vi "Retrieve Number Of Processors From Registry.vi"(8 "error in":errorcluster) -> (0 "error out":errorcluster, 3 "Number Of Cores":i32)   [LabVIEW 2013, in "Win32 Util.lvlib"]
doc: "Query the Windows registry for the number of processors present in the system.\n\nNote: this VI has not been thoroughly tested. It works fine on the developers Quad core."
uses:
  Win32 Util.lvlib
  <vilib>/registry/registry.llb/Registry SAM.ctl
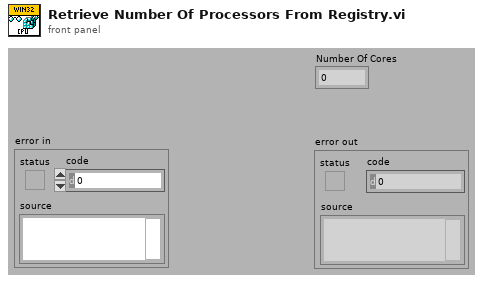
[diagram p1: front panel]
types:
  T1 = typedef "Registry SAM.ctl" = enum32{"KEY_QUERY_VALUE", "KEY_SET_VALUE", "KEY_CREATE_SUB_KEY", "KEY_ENUMERATE_SUB_KEYS", "KEY_NOTIFY", "KEY_CREATE_LINK", "KEY_READ", "KEY_WRITE", "KEY_ALL_ACCESS", "KEY_READ | KEY_WRITE"}
  T2 = typedef "Registry refnum.ctl" = refnum<k1>
  T3 = cluster{"numSubKeys":i32, "maxSubKeyLen":i32, "maxSubKeyClassLen":i32}
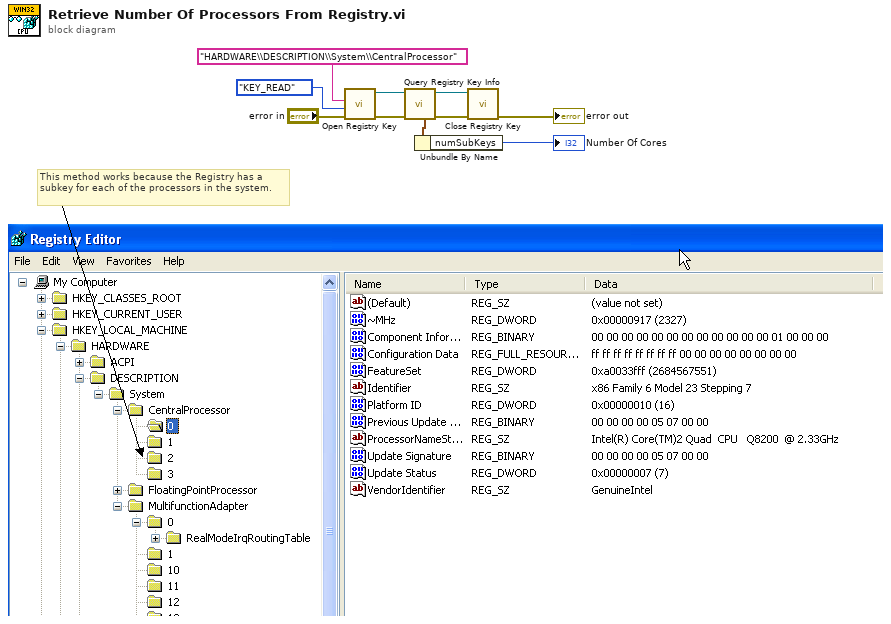
[diagram p0: block diagram]
diagram:
  # "This method works because the Registry has a subkey for each of the processors in the system."
  n1 = call <vilib>:"Open Registry Key.vi"("error in (no error)"="error in", "security access mask (KEY_READ | KEY_WRITE)"=Registry_SAM."KEY_READ", "subkey"="HARDWARE\\DESCRIPTION\\System\\CentralProcessor") -> ("error out"=w6:errorcluster, "refnum out"=w9:T2)  [unwired: 1 in, 6 out]
  n2 = call <vilib>:"Query Registry Key Info.vi"("error in (no error)"=w6, "refnum"=w9) -> ("error out"=w5:errorcluster, "refnum out"=w8:T2, "subkey info"=w7:T3)  [unwired: 7 out]
  n3 = Unbundle By Name(w7) -> ("numSubKeys"=→"Number Of Cores":i32)
  n4 = call <vilib>:"Close Registry Key.vi"("error in (no error)"=w5, "refnum"=w8) -> ("error out"=→"error out":errorcluster)  [unwired: 5 out]
